vi "subDFD_Load Busy VI.vi"() -> (0 "error out":errorcluster, 3 "Busy vi reference":refnum<vi>)   [LabVIEW 2017]
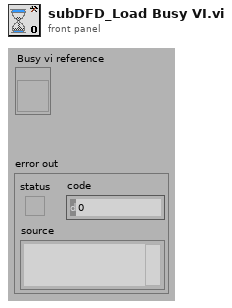
[diagram p1: front panel]
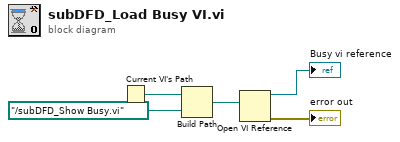
[diagram p0: block diagram]
diagram:
  n1 = Current VI's Path() -> (path=w5:path)
  n2 = Build Path(base path=w5, name or relative path=path "../subDFD_Show Busy.vi") -> (appended path=w4:path)
  n3 = Open VI Reference(vi path=w4) -> (vi reference=→"Busy vi reference":refnum<vi>, error out=→"error out":errorcluster)  [unwired: 1 in, 4 out]
